vi "Main_17a.vi"() -> ()   [LabVIEW 2023]
uses:
  Cluster_Node.ctl
  Cluster_Point Data.ctl
  ENUM_Direction.ctl
panel:
  out "Num Array 2":i32[][](array[numeric])
  out "Num Array":i32[][](array[numeric])
  out "Answer":u32
  in  "Puzzle":string="233233113311241121234343343214331245213144241553252132155521311253254232542552344353534322253245553142552222531524412411331424111421312212221\n312332233233121234131122114442251122232145423545335523152214246544444232542642636454111211355541425253155441432121511431224122231421212331313\n232122343233344323333222224215141321444135531541531234453364436333244664223335653336254441535433321225333134321355351432341342431342413121323\n131222114244332211432122232142231525435152314444141422526445623462354266446443326254353463635254334131221553134122443334422121441341112322323\n23313321141144114331344211315345..."
  in  "Example":string="2413432311323\n3215453535623\n3255245654254\n3446585845452\n4546657867536\n1438598798454\n4457876987766\n3637877979653\n4654967986887\n4564679986453\n1224686865563\n2546548887735\n4322674655533"
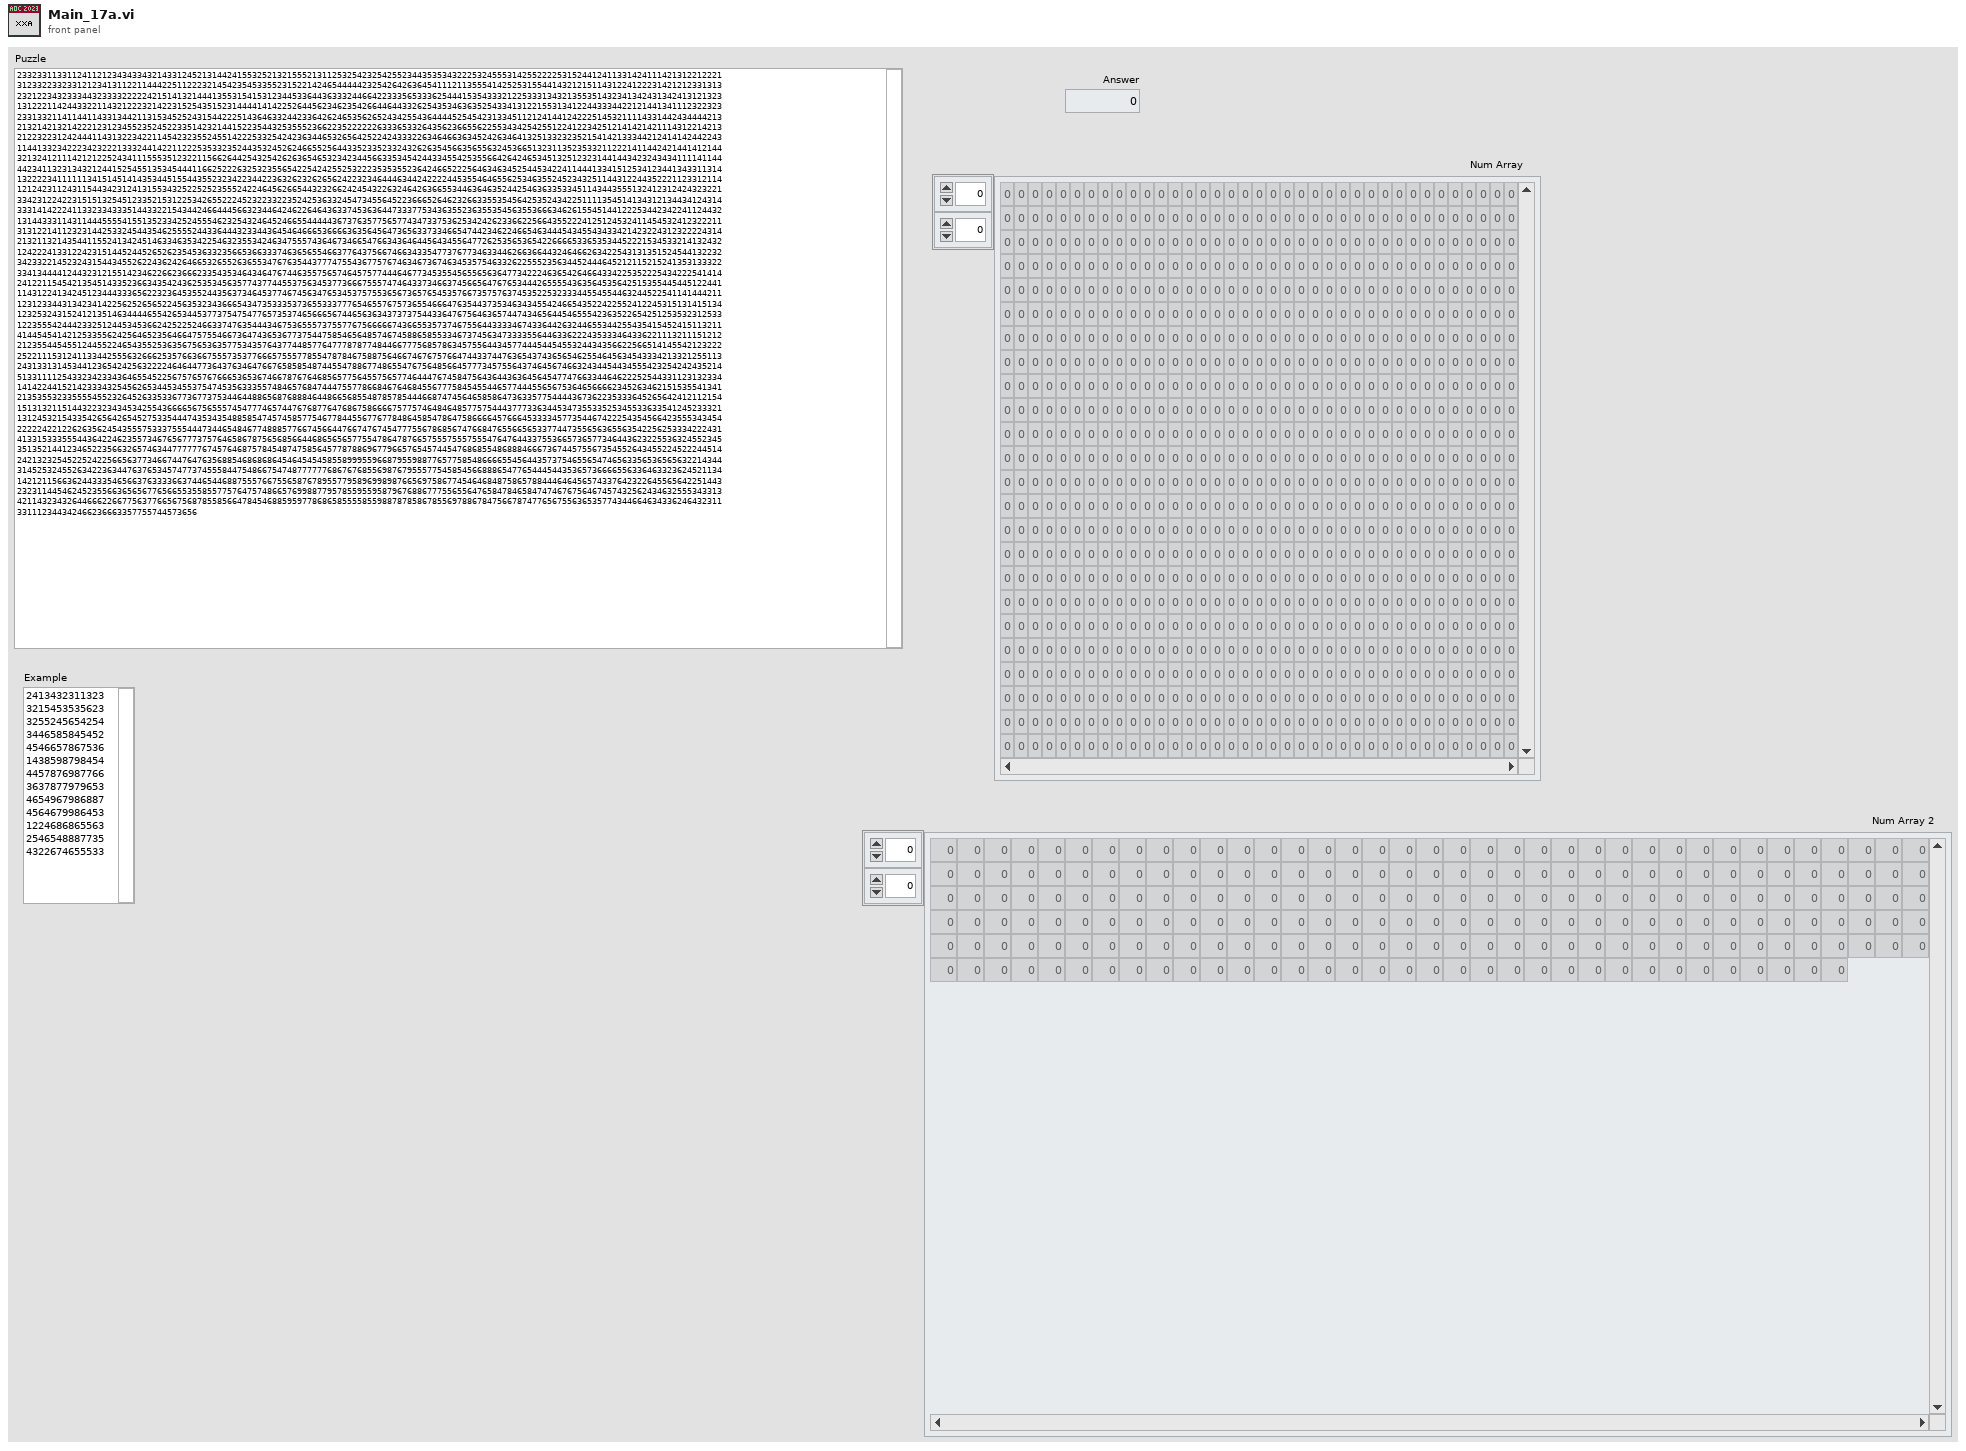
[diagram p1: front panel]
types:
  T1 = typedef "Cluster_Node.ctl" = cluster{"Row":i32, "Column":i32}
  T2 = typedef "Cluster_Point Data.ctl" = cluster{"score":i32, "Direction":T3, "count":i32}
  T3 = typedef "ENUM_Direction.ctl" = enum16{"Up", "Left", "Down", "Right"}
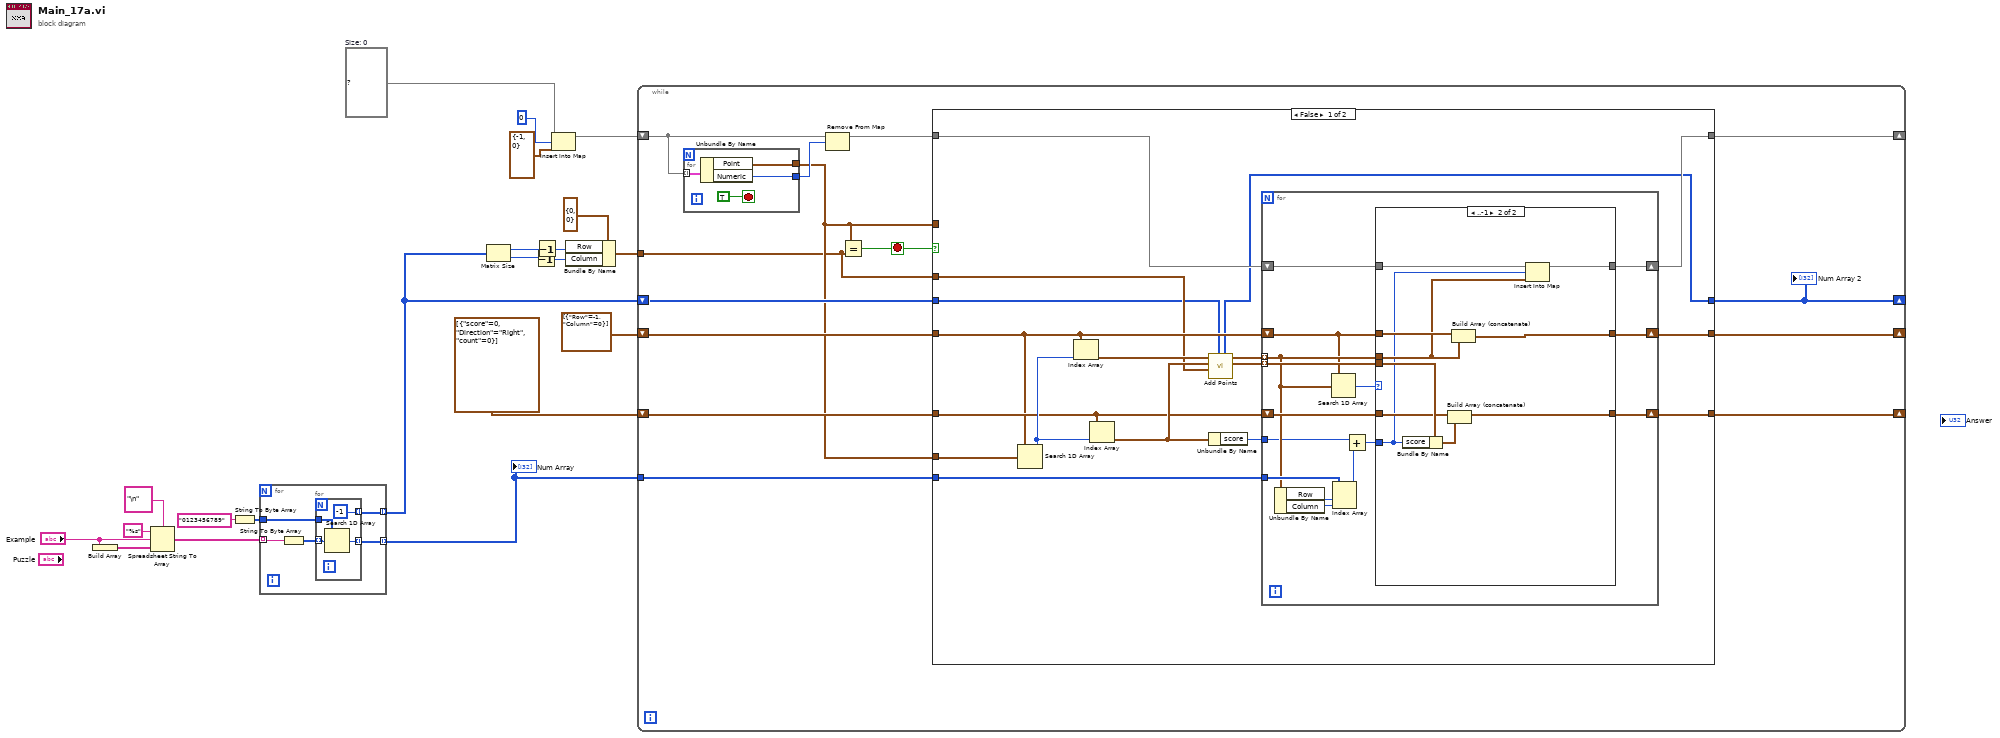
[diagram p0: block diagram]
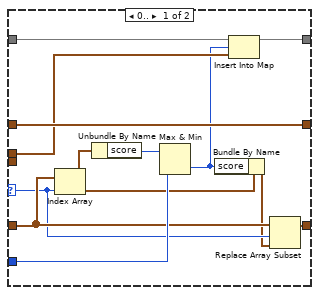
[diagram p2: hidden frame]
diagram:
  w12 = map{i32, T1} {}  # Size: 0
  n1 = Build Array("Example") -> (w21:string[])
  n2 = Spreadsheet String To Array(delimiter (Tab)="\n", format string="%s", spreadsheet string="Example", array type (2D Dbl)=w21) -> (array=w17:string[])
  n3 = String To Byte Array(string="0123456789" ("format string")) -> (unsigned byte array=w15:u8[])
  n4 = for {
    tunnel: w17 -> [w26] mode=indexing
    tunnel: w15 -> [w25]
    tunnel: [w23] -> w14 mode=indexing
    tunnel: [w22] -> w7 mode=indexing
    n5 = String To Byte Array(string=w26) -> (unsigned byte array=w24:u8[])
    n6 = for {
      tunnel: w25 -> [w29]
      tunnel: w24 -> [w30] mode=indexing
      tunnel: [w28] -> w23 mode=indexing
      tunnel: [-1] -> w22 mode=indexing
      n7 = Search 1D Array(1D array=w29, element=w30) -> (index of element=w28:i32)  [unwired: 1 in]
    }
  }
  "Num Array" <- w14
  n8 = Matrix Size(0:w7) -> (1:w6:i32, 2:w5:i32)
  n9 = Decrement(x=w5) -> (x-1=w2:i32)
  n10 = Decrement(x=w6) -> (x-1=w3:i32)
  n11 = Insert Into Map(map in=w12, key=0, value=T1 {"Row"=-1, "Column"=0} ("Point")) -> (map out=w11:map{i32, T1})  [unwired: 2 out]
  n12 = Bundle By Name(cluster=T1 {"Row"=0, "Column"=0} ("Point"), "Row"=w3, "Column"=w2) -> (w1:T1)
  n13 = while {
    tunnel: w14 -> [w38]
    shift-right: [w36] -> _
    shift-left: T2[] [{"score"=0, "Direction"=enum."Right", "count"=0}] ("Array") -> [w42]
    shift-right: [w37] -> _
    shift-left: T1[] [{"Row"=-1, "Column"=0}] ("Array") -> [w41]
    shift-right: [w39] -> _
    shift-left: w11 -> [w44]
    shift-right: [w34] -> _
    shift-left: w7 -> [w35]
    tunnel: w1 -> [w31]
    stop <- w33 stop-if-true
    n14 = for {
      tunnel: w44 -> [w105] mode=indexing
      tunnel: [w104] -> w32
      tunnel: [w103] -> w43
      stop <- TRUE stop-if-true
      n15 = Unbundle By Name(w105) -> ("Point"=w104:T1, "Numeric"=w103:i32)
    }
    n16 = Remove From Map(10:w43, 11:w44) -> (3:w40:map{i32, T1})  [unwired: 2 out]
    n17 = Equal?(x=w32, y=w31) -> (x = y?=w33:bool)
    n18 = case shown="False" w33 {
      tunnel: w42 -> [w55 w99]
      tunnel: w41 -> [w54 w100]
      tunnel: w40 -> [w53 w102]
      tunnel: [w52 w102] -> w39
      tunnel: w38 -> [w51 _]
      tunnel: [w50 w100] -> w37
      tunnel: [w49 w99] -> w36
      tunnel: w35 -> [w46 w101]
      tunnel: [w45 w101] -> w34
      tunnel: w32 -> [w48 _]
      tunnel: w32 -> [_ _]
      tunnel: w31 -> [w47 _]
      frame False {
        n19 = Search 1D Array(1D array=w54, element=w48) -> (index of element=w61:i32)  [unwired: 1 in]
        n20 = Index Array(array=w54, index=w61) -> (element=w60:T1)
        n21 = Index Array(array=w55, index=w61) -> (element=w57:T2)
        n22 = call "Add Points.vi"("Num Array Out"=w46, "Max Point"=w47, "Point Data"=w57, "Point"=w60) -> ("Data Array Out"=w58:T2[], "Point Array Out"=w59:T1[], "Num Array Out 2"=w45:i32[][])  [unwired: 5 in]
        n23 = Unbundle By Name(w57) -> ("score"=w56:i32)
        n24 = for {
          tunnel: w59 -> [w72] mode=indexing
          tunnel: w58 -> [w75] mode=indexing
          tunnel: w56 -> [w68]
          shift-right: [w65] -> w49
          shift-left: w55 -> [w74]
          shift-right: [w64] -> w50
          shift-left: w54 -> [w66]
          shift-right: [w62] -> w52
          shift-left: w53 -> [w63]
          tunnel: w51 -> [w73]
          n25 = Unbundle By Name(w72) -> ("Row"=w71:i32, "Column"=w70:i32)
          n26 = Search 1D Array(1D array=w66, element=w72) -> (index of element=w76:i32)  [unwired: 1 in]
          n27 = Index Array(array=w73, index (row)=w71, index (col)=w70) -> (element=w69:i32)
          n28 = Add(x=w68, y=w69) -> (x+y=w67:i32)
          n29 = case shown="..-1" w76 {
            selector: w76 -> [w81 _]
            tunnel: w75 -> [_ w98]
            tunnel: w72 -> [w78 w90]
            tunnel: w66 -> [w86 w97]
            tunnel: w74 -> [w83 w95]
            tunnel: w67 -> [w84 w89]
            tunnel: [w82 w94] -> w65
            tunnel: [w86 w93] -> w64
            tunnel: w63 -> [w88 w92]
            tunnel: [w87 w91] -> w62
            frame 0.. {
              n30 = Index Array(array=w83, index=w81) -> (element=w80:T2)
              n31 = Unbundle By Name(w80) -> ("score"=w85:i32)
              n32 = Max & Min(x=w85, y=w84) -> (min(x,y)=w77:i32)  [unwired: 1 out]
              n33 = Bundle By Name(cluster=w80, "score"=w77) -> (w79:T2)
              n34 = Insert Into Map(map in=w88, key=w77, value=w78) -> (map out=w87:map{i32, T1})  [unwired: 2 out]
              n35 = Replace Array Subset(array=w83, new element=w79, index=w81) -> (w82:T2[])
            }
            frame ..-1 {
              n36 = Bundle By Name(cluster=w98, "score"=w89) -> (w96:T2)
              n37 = Build Array (concatenate)(w95, w96) -> (w94:T2[])
              n38 = Build Array (concatenate)(w97, w90) -> (w93:T1[])
              n39 = Insert Into Map(map in=w92, key=w89, value=w90) -> (map out=w91:map{i32, T1})  [unwired: 2 out]
            }
          }
        }
      }
      frame True {
      }
    }
    "Num Array 2" <- w34
  }
